vi "Channel Source Power Set Correction On.vi"(7 "Val (Off)":bool, 8 "error in (no error)":errorcluster {"code" format="%.0x"}, 9 "PortVal":i32 format="%.0g", 10 "RepCapIdentifier":string, 11 "instrument handle":refnum<k15>) -> (0 "error out":errorcluster {"code" format="%.0x"}, 3 "instrument handle out":refnum<k15>)   [LabVIEW 2014, in "Agilent NA.lvlib"]
doc: "Enables and disables source power correction for the specified port on the specified channel."
uses:
  Agilent NA.lvlib
  AgNA.dll
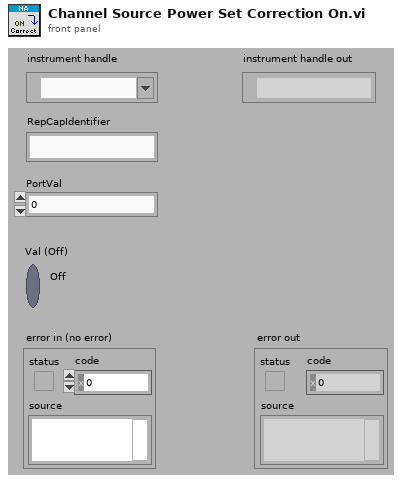
[diagram p1: front panel]
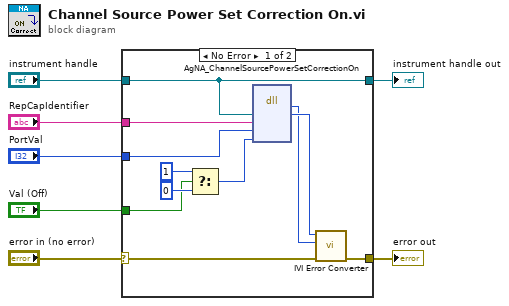
[diagram p0: block diagram]
diagram:
  n1 = case shown="No Error" "error in (no error)" {
    selector: "error in (no error)" -> [w16 w20]
    tunnel: [w15 w20] -> w7
    tunnel: "RepCapIdentifier" -> [w14 _]
    tunnel: "PortVal" -> [w13 _]
    tunnel: [w12 w19] -> w3
    tunnel: "instrument handle" -> [w12 w19]
    tunnel: "Val (Off)" -> [w8 _]
    frame No Error {
      n2 = Select(t=u16 1, s=w8, f=u16 0) -> (s? t:f=w10:u16)
      n3 = dll-call lib="AgNA**.dll" fn="AgNA_ChannelSourcePowerSetCorrectionOn"("Vi"=w12, "RepCapIdentifier"=w14, "PortVal"=w13, "Val"=w10) -> (w17:i32, "Vi"=w18:u32)  [unwired: 6 in, 2 out]
      n4 = call "IVI Error Converter.vi"("error in (no error)"=w16, "IVI error code (0)"=w17, "instrument handle"=w18) -> ("error out"=w15:errorcluster)  [unwired: 7 in, 1 out]
    }
    frame Error {
    }
  }
  "error out" <- w7
  "instrument handle out" <- w3
